vi "Read NumAvg.vi"(8 "error in (no error)":errorcluster, 11 "SEDSpectrometer in":refnum<class "FiberSpectrograph.lvclass">) -> (0 "error out":errorcluster, 2 "NumAvg":u32=1 caption="Number of averages", 3 "SEDSpectrometer out":refnum<class "FiberSpectrograph.lvclass">)   [LabVIEW 2016, in "FiberSpectrograph.lvclass"]
uses:
  FiberSpectrograph.lvclass
  FiberSpectrograph.lvclass/FiberSpectrograph.ctl
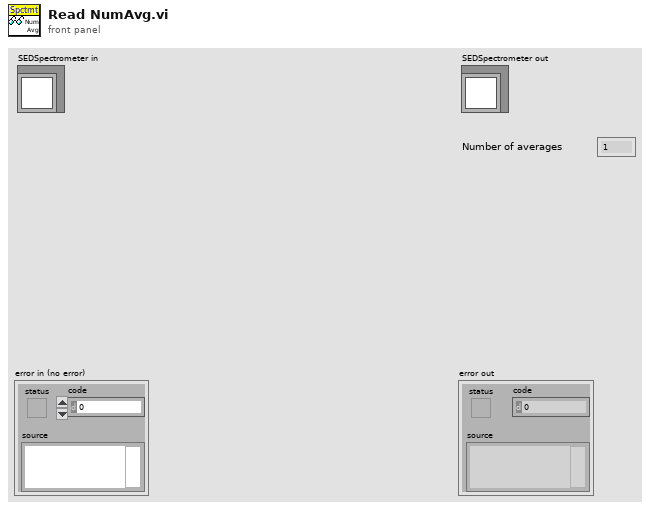
[diagram p1: front panel]
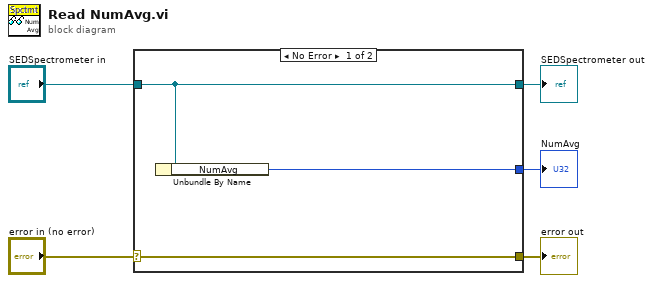
[diagram p0: block diagram]
diagram:
  n1 = case shown="No Error" "error in (no error)" {
    selector: "error in (no error)" -> [w8 w9]
    tunnel: [w8 w9] -> w4
    tunnel: [w7 w10] -> w2
    tunnel: "SEDSpectrometer in" -> [w7 w10]
    tunnel: [w6 _] -> w1
    frame No Error {
      n2 = Unbundle By Name(w7) -> ("NumAvg"=w6:u32)
    }
    frame Error {
    }
  }
  "error out" <- w4
  "SEDSpectrometer out" <- w2
  "NumAvg" <- w1
